vi "subscribeToDataType.vi"(7 "ExplodeContainer (F)":bool, 8 "error in":errorcluster, 9 "ObservableData":variant, 11 "ObserverClass in":refnum<class "ObserverClass.lvclass">) -> (0 "error out":errorcluster, 1 "ObservableValue":variant[](array[variant]), 2 "ObservableName":string[](array[string]), 3 "ObserverClass out":refnum<class "ObserverClass.lvclass">)   [LabVIEW 2025, in "ObserverClass.lvlib" / "ObserverClass.lvclass"]
doc: "Subscribe the Observable Data Type and Name for the current Observer Class istance.\nA List of Observable Name and Data Type can be obtained from a Cluster or a LV Class."
uses:
  ObserverClass.lvclass
  ObserverClass.lvlib
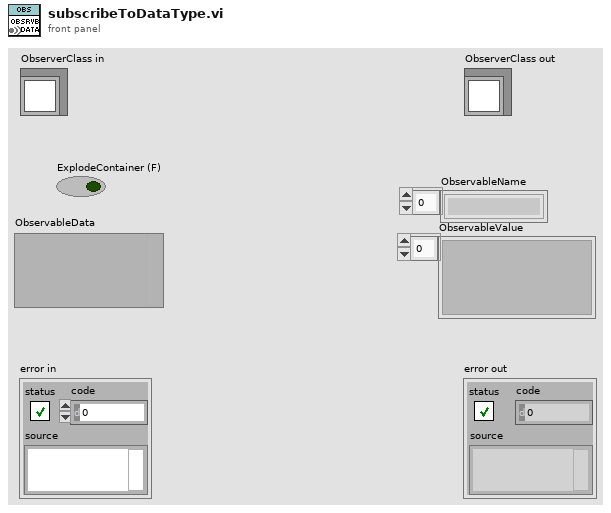
[diagram p1: front panel]
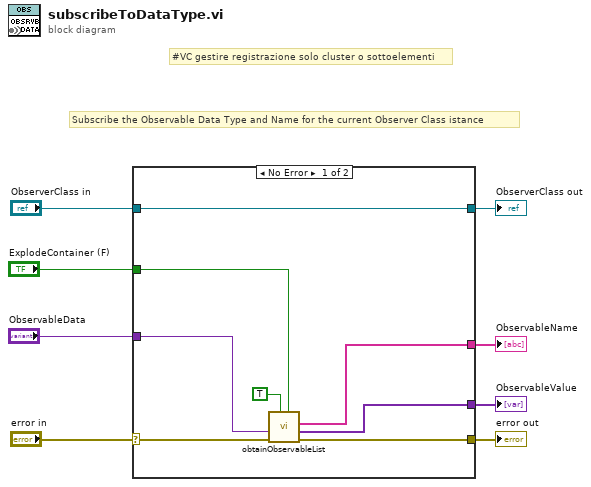
[diagram p0: block diagram]
diagram:
  # "#VC gestire registrazione solo cluster o sottoelementi"
  # "Subscribe the Observable Data Type and Name for the current Observer Class istance"
  n1 = case shown="No Error" "error in" {
    selector: "error in" -> [w16 w18]
    tunnel: [w15 w18] -> w7
    tunnel: [w13 w17] -> w5
    tunnel: "ObserverClass in" -> [w13 w17]
    tunnel: "ObservableData" -> [w14 _]
    tunnel: [w12 _] -> w3
    tunnel: [w11 _] -> w2
    tunnel: "ExplodeContainer (F)" -> [w9 _]
    frame No Error {
      n2 = call "obtainObservableList.vi"("ExplodeContainer (F)"=w9, "AllHierarchy (T)"=TRUE, "error in"=w16, "ObservableData"=w14) -> ("error out"=w15:errorcluster, "ObservableValue"=w11:variant[], "ObservableName"=w12:string[])  [unwired: 5 in]
    }
    frame Error {
    }
  }
  "error out" <- w7
  "ObserverClass out" <- w5
  "ObservableName" <- w3
  "ObservableValue" <- w2
